vi "oa_Get CIC Decimation Filter Coefficients.vi"(6 "CIC stages":i32[](array[numeric])=[4, 6, 8], 7 "reset? (True)":bool=TRUE, 8 "alias protect in final transition":bool, 9 "stop band attenuation":u16(ring) items=["72 dB", "96 dB", "120 dB"], 11 "decimation/interpolation factor":i32=16) -> (0 "delay":i32, 1 "lp filter settings":T1={"coefficients"=[], "factor"=1} {"coefficients" format="%.2f"}, 2 "compensation filter settings":T1={"coefficients"=[], "factor"=1} {"coefficients" format="%.2f"}, 3 "CIC Settings":cluster{"Numeric":i32, i32, i32}, 4 "interpolation factor":i32)   [LabVIEW 2017, in "SoundVib_Resampling.lvlib"]
uses:
  <vilib>/addons/Sound and Vibration/Order Analysis/Resample Order Tracking/SoundVib_Resampling.lvlib
  <vilib>/addons/_NISVFA/_Shared subVIs/Controls/OAT Decimation Filter.ctl
  <vilib>/addons/Sound and Vibration/Order Analysis/Resample Order Tracking/SubVIs/oa_Calculate Delay of CIC Decimation Interpolation Filter.vi
  <vilib>/addons/Sound and Vibration/Order Analysis/Resample Order Tracking/SubVIs/oa_Create CIC Compensation Filter.vi
  <vilib>/addons/Sound and Vibration/Order Analysis/Resample Order Tracking/SubVIs/oa_Create CIC LP Truncation Filter.vi
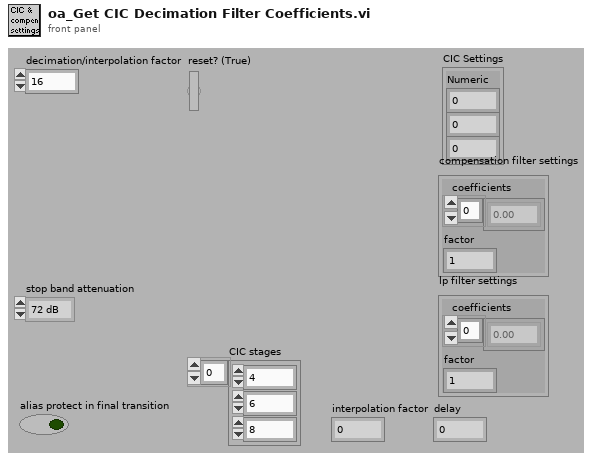
[diagram p1: front panel]
types:
  T1 = typedef "OAT Decimation Filter.ctl" = cluster{"coefficients":dbl[], "factor":i32}
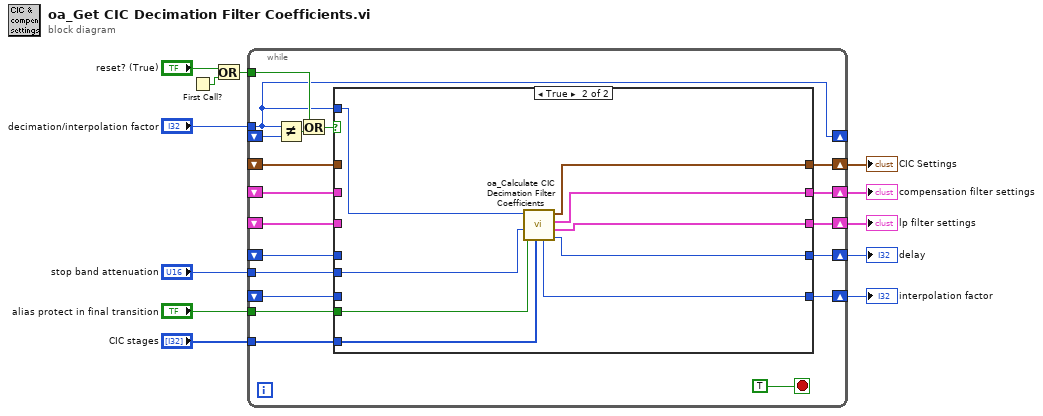
[diagram p0: block diagram]
diagram:
  n1 = First Call?() -> (First Call?: T/F=w12:bool)
  n2 = Or(x="reset? (True)", y=w12) -> (x .or. y?=w10:bool)
  n3 = while {
    tunnel: w10 -> [w29]
    shift-right: [w16] -> _
    shift-left: _ -> [w31]
    tunnel: "decimation/interpolation factor" -> [w16]
    shift-right: [w26] -> w7
    shift-left: _ -> [w24]
    shift-right: [w25] -> w6
    shift-left: _ -> [w23]
    shift-right: [w22] -> w8
    shift-left: _ -> [w21]
    shift-right: [w20] -> w5
    shift-left: _ -> [w19]
    tunnel: "stop band attenuation" -> [w18]
    tunnel: "alias protect in final transition" -> [w17]
    shift-right: [w15] -> w2
    shift-left: _ -> [w14]
    tunnel: "CIC stages" -> [w13]
    stop <- TRUE stop-if-true
    n4 = Not Equal?(x=w16, y=w31) -> (x != y?=w30:bool)
    n5 = Or(x=w29, y=w30) -> (x .or. y?=w28:bool)
    n6 = case shown="True" w28 {
      tunnel: w16 -> [_ w45]
      tunnel: [w36 w38] -> w26
      tunnel: [w35 w37] -> w25
      tunnel: w24 -> [w36 _]
      tunnel: w23 -> [w35 _]
      tunnel: [w34 w40] -> w22
      tunnel: w21 -> [w34 _]
      tunnel: [w33 w41] -> w20
      tunnel: w19 -> [w33 _]
      tunnel: w18 -> [_ w44]
      tunnel: w17 -> [_ w43]
      tunnel: [w32 w39] -> w15
      tunnel: w14 -> [w32 _]
      tunnel: w13 -> [_ w42]
      frame False {
      }
      frame True {
        n7 = call <vilib>:"oa_Calculate CIC Decimation Filter Coefficients.vi"("CIC stages"=w42, "alias protect in final transition"=w43, "stop band attenuation"=w44, "decimation/interpolation factor"=w45) -> ("delay"=w39:i32, "lp filter settings"=w37:T1, "compensation filter settings"=w38:T1, "CIC Settings"=w40:cluster{"Numeric":i32, i32, i32}, "interpolation factor"=w41:i32)  [unwired: 3 in]
      }
    }
  }
  "CIC Settings" <- w8
  "compensation filter settings" <- w7
  "lp filter settings" <- w6
  "interpolation factor" <- w5
  "delay" <- w2
